vi "Set Center and Radius.vi"(9 "Radius":u16=1, 10 "Point.lvclass":refnum<class "Point.lvclass">, 11 "Circle in":refnum<class "Circle.lvclass">) -> (3 "Circle out":refnum<class "Circle.lvclass">)   [LabVIEW 2018, in "Circle.lvclass"]
doc: "Set center point and radius for the circle."
uses:
  Circle.lvclass
  e:/builds/penguin/labview/branches/2018/dev/dist64/examples/Object-Oriented Programming/Graphics/Graphic/Graphic.lvclass
  Point/Point.lvclass
  Circle.lvclass/Circle.ctl
  Graphic/Graphic.lvclass
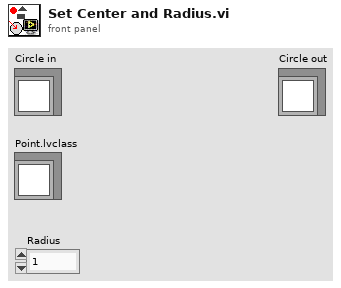
[diagram p1: front panel]
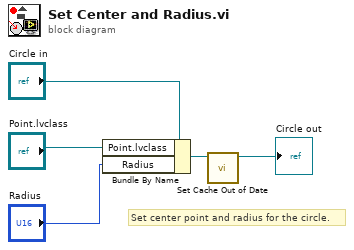
[diagram p0: block diagram]
diagram:
  # "Set center point and radius for the circle."
  n1 = Bundle By Name(cluster="Circle in", "Point.lvclass"="Point.lvclass", "Radius"="Radius") -> (w2:refnum<class "Circle.lvclass">)
  n2 = call "Set Cache Out of Date.vi"("Graphic.lvclass"=w2) -> ("Graphic.lvclass out"=→"Circle out":refnum<class "Circle.lvclass">)  [unwired: 10 in]
